vi "LVFunction_Imop_Compute_SlopeFromCoef.vi"(0 "HasoSlopes.lvclass":refnum<class "HasoSlopes.lvclass">, 5 "ComputePhaseSet":refnum<class "ComputePhaseSet.lvclass">, 7 "ModalCoef.lvclass":refnum<class "ModalCoef.lvclass">, 11 "error IO":errorcluster) -> (4 "HasoSlopes.lvclass":refnum<class "HasoSlopes.lvclass">, 6 "ComputePhaseSet (dup)":refnum<class "ComputePhaseSet.lvclass">, 8 "ModalCoef.lvclass (dup)":refnum<class "ModalCoef.lvclass">, 15 "error IO out":errorcluster)   [LabVIEW 2020]
doc: "Compute slopes from modal coefficients that represent them in a given basis of\npolynomials provided by ComputePhaseSet. Modal coeffs must have a projection\npupil set in their preferences.\n\n<B>ComputePhaseSetIn</B> : ComputePhaseSet object.\n<B>ComputePhaseSetOut</B> : ComputePhaseSet object.\n<B>ModalCoeffs</B> : ModalCoef object.\n<B>HasoSlopes</B> : HasoSlopes object."
uses:
  ModalCoef.lvclass
  HasoSlopes.lvclass
  ComputePhaseSet.lvclass
  LVClass_HasoSlopes Read HasoSlopes _ property.vi
  LVClass_ModalCoef Read ModalCoef.vi
  LVClass_ComputePhaseSet Read ComputePhaseSet.vi
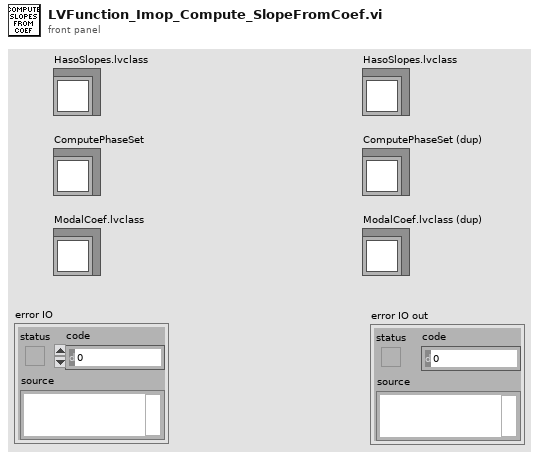
[diagram p1: front panel]
types:
  T1 = typedef "ClassID.ctl" = i64
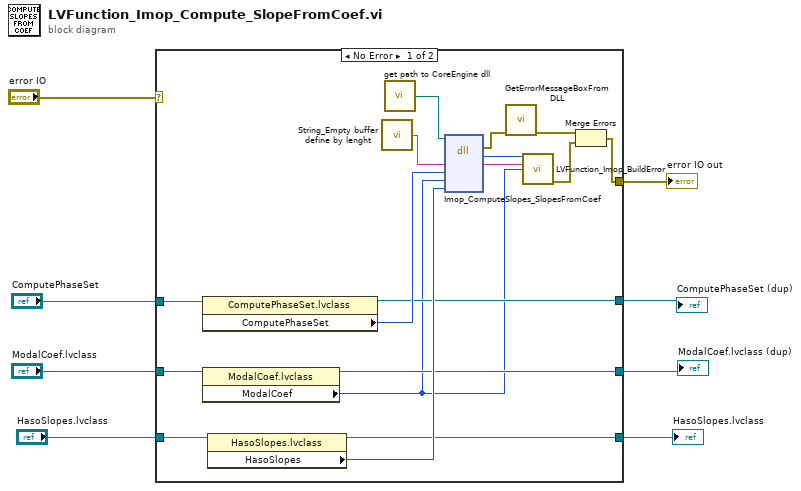
[diagram p0: block diagram]
diagram:
  n1 = case shown="No Error" "error IO" {
    selector: "error IO" -> [_ w29]
    tunnel: [w13 w29] -> w7
    tunnel: "ComputePhaseSet" -> [w20 w27]
    tunnel: "ModalCoef.lvclass" -> [w19 w26]
    tunnel: "HasoSlopes.lvclass" -> [w18 w28]
    tunnel: [w16 w28] -> w5
    tunnel: [w11 w27] -> w2
    tunnel: [w10 w26] -> w1
    frame No Error {
      n2 = property class="ComputePhaseSet.lvclass"(reference=w20) -> (reference out=w11:refnum<class "ComputePhaseSet.lvclass">, "ComputePhaseSet"=w12:T1)  [unwired: 1 in, 1 out]
      n3 = property class="ModalCoef.lvclass"(reference=w19) -> (reference out=w10:refnum<class "ModalCoef.lvclass">, "ModalCoef"=w9:T1)  [unwired: 1 in, 1 out]
      n4 = property class="HasoSlopes.lvclass"(reference=w18) -> (reference out=w16:refnum<class "HasoSlopes.lvclass">, "HasoSlopes"=w17:T1)  [unwired: 1 in, 1 out]
      n5 = call "String_Empty buffer define by lenght.vi"() -> ("Empty buffer"=w23:string)  [unwired: 1 in]
      n6 = call "get path to CoreEngine dll.vi"() -> ("path to wavekit library"=w22:path)  [unwired: 14 in, 1 out]
      n7 = dll-call lib="D:/FLE/0.Code/CoreEngine4_Suite/LV2011_interface/DLLs/c_interface_vc100.dll" fn="Imop_ComputeSlopes_SlopesFromCoef"(path in=w22, "message"=w23, "computePhaseSet"=w12, "ModalCoeffs"=w9, "HasoSlopes"=w17) -> (error out=w21:errorcluster, "return type"=w25:i32, "message"=w24:string)  [unwired: 5 in, 1 out]
      n8 = call "GetErrorMessageBoxFromDLL.vi"("error IN"=w21) -> ("error OUT"=w15:errorcluster)  [unwired: 10 in]
      n9 = call "LVFunction_Imop_BuildError.vi"("code"=w25, "String to Prepend to source (\"\")"=w24, "Adresse"=w9) -> ("error out"=w14:errorcluster)  [unwired: 12 in]
      n10 = Merge Errors(w15, w14) -> (w13:errorcluster)
    }
    frame Error {
    }
  }
  "error IO out" <- w7
  "ModalCoef.lvclass (dup)" <- w1
  "HasoSlopes.lvclass" <- w5
  "ComputePhaseSet (dup)" <- w2
